vi "EditPatientDataInfoArmPressure-Kamronn-Medtech.vi"() -> (3 "Save?":bool)   [LabVIEW 2013, in "main.lvlib"]
uses:
  main.lvlib
panel:
  in  "CancelEditPressureBtn":bool
  in  "SavePressureBtn":bool
  in  "LeftArray":T1(array[cluster])
  in  "RightArray":T1(array[cluster])
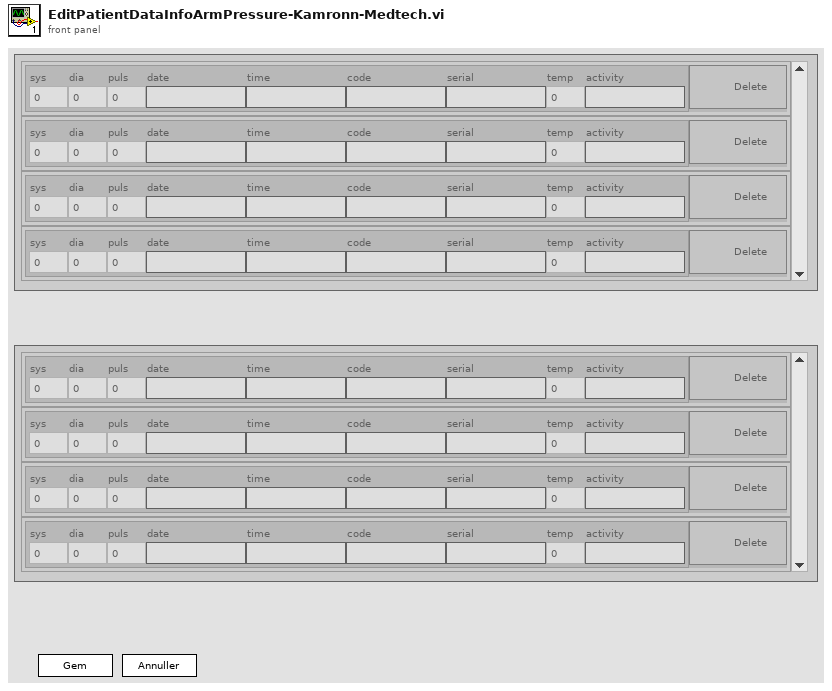
[diagram p1: front panel]
types:
  T1 = cluster{"data":cluster{"sys":dbl, "dia":dbl, "puls":dbl, "date":string, "time":string, "code":string, "serial":string, "temp":dbl, "activity":string}, "Delete Button":bool}[]
  T2 = cluster{"sys":dbl, "dia":dbl, "puls":dbl, "date":string, "time":string, "code":string, "serial":string, "temp":dbl, "activity":string}[]
  T3 = cluster{"data":cluster{"sys":dbl, "dia":dbl, "puls":dbl, "date":string, "time":string, "code":string, "serial":string, "temp":dbl, "activity":string}, "Delete":bool}
  T4 = cluster{"sys":dbl, "dia":dbl, "puls":dbl, "date":string, "time":string, "code":string, "serial":string, "temp":dbl, "activity":string}
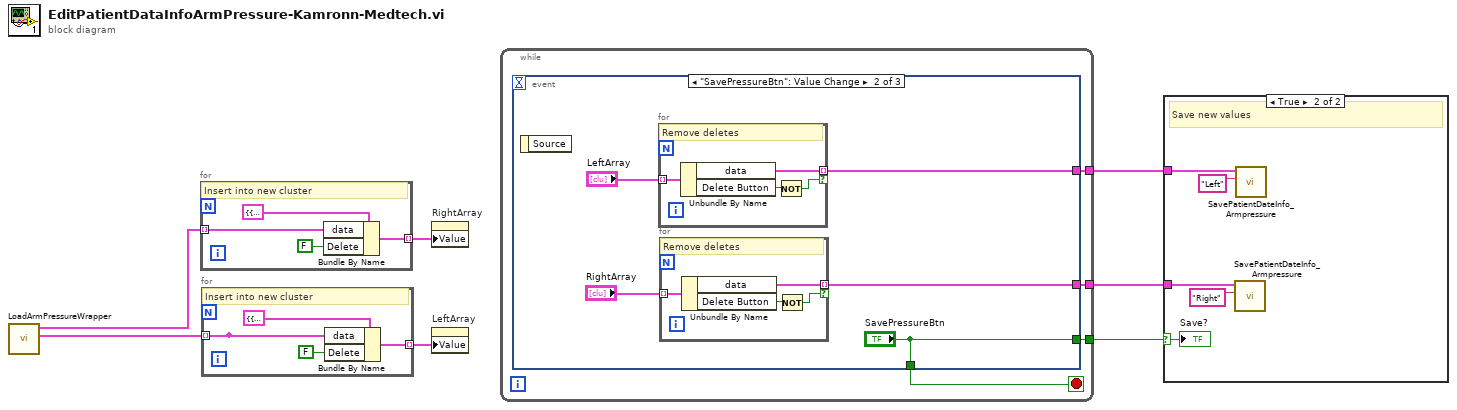
[diagram p0: block diagram]
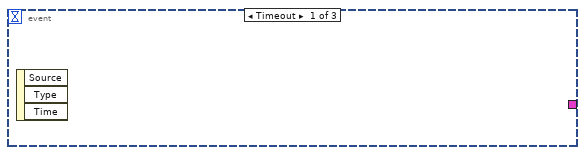
[diagram p3: hidden frame]
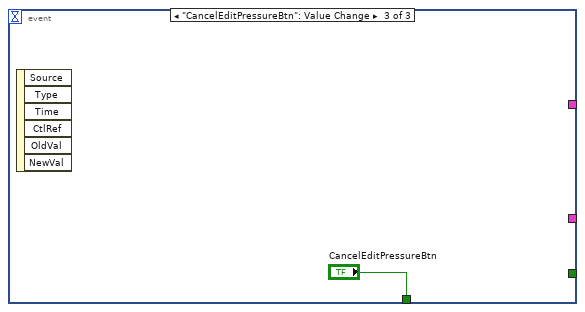
[diagram p4: hidden frame]
diagram:
  n1 = call "LoadArmPressureWrapper.vi"() -> ("Armpressure Left"=w5:T2, "Armpressure Right"=w7:T2)  [unwired: 9 in, 1 out]
  n2 = for {
    tunnel: w7 -> [w8] mode=indexing
    tunnel: [w10] -> w6 mode=indexing
    # "Insert into new cluster"
    n3 = Bundle By Name(cluster=T3 {"data"={"sys"=0.0, "dia"=0.0, "puls"=0.0, "date"="", "time"="", "code"="", "serial"="", "temp"=0.0, "activity"=""}, "Delete"=FALSE}, "data"=w8, "Delete"=FALSE) -> (w10:T3)
  }
  n4 = for {
    tunnel: [w12] -> _ mode=indexing
    tunnel: [w14] -> w4 mode=indexing
    tunnel: w5 -> [w12] mode=indexing
    # "Insert into new cluster"
    n5 = Bundle By Name(cluster=T3 {"data"={"sys"=0.0, "dia"=0.0, "puls"=0.0, "date"="", "time"="", "code"="", "serial"="", "temp"=0.0, "activity"=""}, "Delete"=FALSE}, "data"=w12, "Delete"=FALSE) -> (w14:T3)
  }
  n6 = property on="RightArray" class="Arr"("Value"=w6) -> ()  [unwired: 2 in, 2 out]
  n7 = property on="LeftArray" class="Arr"("Value"=w4) -> ()  [unwired: 2 in, 2 out]
  n8 = while {
    tunnel: [w18] -> w3
    tunnel: [w17] -> w2
    tunnel: [w16] -> w1
    stop <- w19 stop-if-true
    n9 = event shown="[1] \"SavePressureBtn\": Value Change" {
      selector: _ -> [_ _ _]
      dyn-events: _ -> [_ _ _]
      timeout: _ -> [_ _ _]
      tunnel: [_ "SavePressureBtn" "CancelEditPressureBtn"] -> w19
      tunnel: [_ w22 _] -> w18
      tunnel: [_ "SavePressureBtn" _] -> w17
      tunnel: [_ w20 _] -> w16
      event Timeout {
        n10 = event-data() -> ()  [unwired: 1 in, 3 out]
      }
      event "SavePressureBtn": Value Change {
        n11 = event-data() -> ()  [unwired: 1 in, 1 out]
        n12 = for {
          tunnel: "LeftArray" -> [w32] mode=indexing
          tunnel: [w31] -> w22 mode=indexing if=w29
          # "Remove deletes"
          n13 = Unbundle By Name(w32) -> ("data"=w31:T4, "Delete Button"=w30:bool)
          n14 = Not(x=w30) -> (.not. x?=w29:bool)
        }
        n15 = for {
          tunnel: "RightArray" -> [w28] mode=indexing
          tunnel: [w27] -> w20 mode=indexing if=w25
          # "Remove deletes"
          n16 = Unbundle By Name(w28) -> ("data"=w27:T4, "Delete Button"=w26:bool)
          n17 = Not(x=w26) -> (.not. x?=w25:bool)
        }
      }
      event "CancelEditPressureBtn": Value Change {
        n18 = event-data() -> ()  [unwired: 1 in, 6 out]
      }
    }
  }
  n19 = case shown="True" w2 {
    selector: w2 -> [_ w34]
    tunnel: w3 -> [_ w38]
    tunnel: w1 -> [_ w37]
    frame False {
    }
    frame True {
      # "Save new values"
      n20 = call "SavePatientDateInfo_Armpressure.vi"("Side(Left/Right)"="Right", "Pressure"=w37) -> ()  [unwired: 9 in, 1 out]
      n21 = call "SavePatientDateInfo_Armpressure.vi"("Side(Left/Right)"="Left", "Pressure"=w38) -> ()  [unwired: 9 in, 1 out]
      "Save?" <- w34
    }
  }
